vi "Motor_Speed.vi"() -> ()   [LabVIEW 2024]
panel:
  out "In Range?":bool
  out "Meter":dbl(knob) scale=0.0..100.0
  out "Numeric":dbl
  in  "Knob":dbl(knob) scale=0.0..100.0
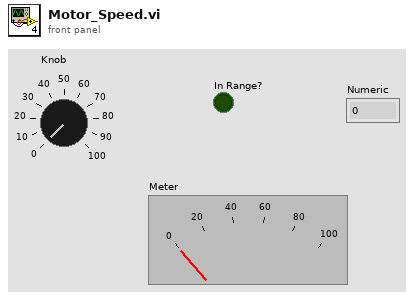
[diagram p1: front panel]
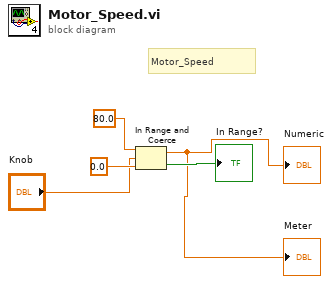
[diagram p0: block diagram]
diagram:
  # "Motor_Speed"
  n1 = In Range and Coerce(upper limit=80.0, x="Knob", lower limit=0.0) -> (coerced(x)=→"Numeric" →"Meter":dbl, In Range?=→"In Range?":bool)
